vi "3_Case_loop.vi"() -> ()   [LabVIEW 2019]
uses:
  Instance           1 17Saved   Case_loop .vi
panel:
  in  "Enum":T1(ring) caption="Funkcja"
  out "?":bool
  out "?":bool
  out "?":bool=TRUE
  out "?":bool
  out "?":bool
  out "?":bool
  in  "Opóznienie [s]":dbl=0.009999999999999997 caption="Delay Time (s)" min=0.0 step=0.01 format="%#.2g"
  out "Waveform Chart":dynamicdata(graph)=[{"t0"=timestamp(3254228964.578125 s since 1904-01-01), "dt"=1.0, "Y"=[-0.9998476951563912]}, {"t0"=timestamp(3254228964.578125 s since 1904-01-01), "dt"=1.0, "Y"=[0.0]}]
  out "Numer iteracji":dbl=1709.0
  in  "?":bool
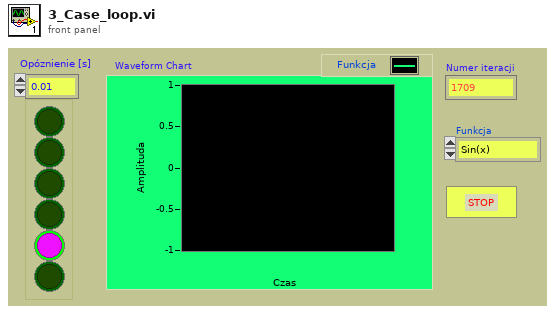
[diagram p1: front panel]
types:
  T1 = enum16{"Sin(x)", "Sin(x)+Cos(x)", "Sin(x)/x", "Sin(x)-Sin(2x)"}
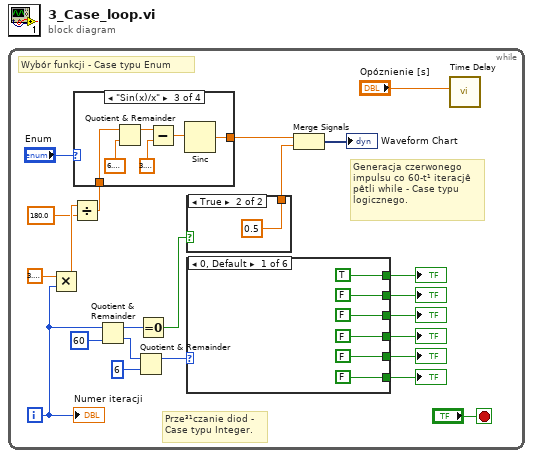
[diagram p0: block diagram]
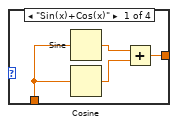
[diagram p2: hidden frame]
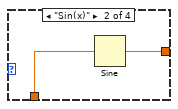
[diagram p3: hidden frame]
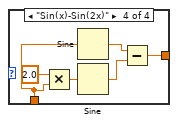
[diagram p4: hidden frame]
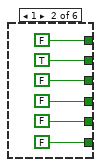
[diagram p5: hidden frame]
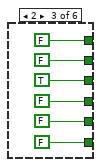
[diagram p6: hidden frame]
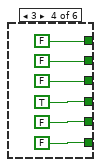
[diagram p7: hidden frame]
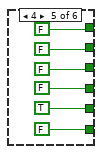
[diagram p8: hidden frame]
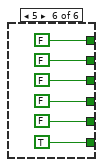
[diagram p9: hidden frame]
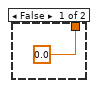
[diagram p10: hidden frame]
diagram:
  n1 = while {
    i -> [w11]
    stop <- "?" stop-if-true
    # "Wybór funkcji - Case typu Enum"
    # "Prze³¹czanie diod -\nCase typu Integer."
    # "Generacja czerwonego\nimpulsu co 60-t¹ iteracjê\npêtli while - Case typu \nlogicznego."
    n2 = Multiply(x=3.141592653589793, y=w11) -> (x*y=w13:dbl)
    n3 = Divide(x=w13, y=180.0) -> (x/y=w1:dbl)
    n4 = case shown="\"Sin(x)/x\"" "Enum" {
      tunnel: [w24 w29 w35 w41] -> w3
      tunnel: w1 -> [w27 w28 w30 w38]
      frame "Sin(x)+Cos(x)" {
        n5 = Sine(x=w27) -> (sin(x)=w25:dbl)
        n6 = Cosine(x=w27) -> (cos(x)=w26:dbl)
        n7 = Add(x=w25, y=w26) -> (x+y=w24:dbl)
      }
      frame "Sin(x)" {
        n8 = Sine(x=w28) -> (sin(x)=w29:dbl)
      }
      frame "Sin(x)/x" {
        n9 = Quotient & Remainder(x=w30, y=6.283185307179586) -> (x-y*floor(x/y)=w33:dbl)  [unwired: 1 out]
        n10 = Subtract(x=w33, y=3.141592653589793) -> (x-y=w31:dbl)
        n11 = Sinc(1:w31) -> (0:w35:dbl)
      }
      frame "Sin(x)-Sin(2x)" {
        n12 = Multiply(x=2.0, y=w38) -> (x*y=w37:dbl)
        n13 = Sine(x=w38) -> (sin(x)=w39:dbl)
        n14 = Sine(x=w37) -> (sin(x)=w40:dbl)
        n15 = Subtract(x=w39, y=w40) -> (x-y=w41:dbl)
      }
    }
    n16 = Quotient & Remainder(x=w11, y=60) -> (x-y*floor(x/y)=w9:i32, floor(x/y)=w8:i32)
    n17 = Quotient & Remainder(x=w8, y=6) -> (x-y*floor(x/y)=w6:i32)  [unwired: 1 out]
    n18 = Equal To 0?(x=w9) -> (x = 0?=w21:bool)
    n19 = case shown="True" w21 {
      tunnel: [0.0 ("x") 0.5 ("y")] -> w2
      frame False {
      }
      frame True {
      }
    }
    n20 = case shown="0, Default" w6 {
      tunnel: [FALSE ("Boolean") FALSE ("Boolean") FALSE ("Boolean") FALSE ("Boolean") FALSE ("Boolean") TRUE ("Boolean")] -> w20
      tunnel: [FALSE ("Boolean") FALSE ("Boolean") FALSE ("Boolean") FALSE ("Boolean") TRUE ("Boolean") FALSE ("Boolean")] -> w19
      tunnel: [FALSE ("Boolean") FALSE ("Boolean") FALSE ("Boolean") TRUE ("Boolean") FALSE ("Boolean") FALSE ("Boolean")] -> w18
      tunnel: [FALSE ("Boolean") FALSE ("Boolean") TRUE ("Boolean") FALSE ("Boolean") FALSE ("Boolean") FALSE ("Boolean")] -> w17
      tunnel: [FALSE ("Boolean") TRUE ("Boolean") FALSE ("Boolean") FALSE ("Boolean") FALSE ("Boolean") FALSE ("Boolean")] -> w16
      tunnel: [TRUE ("Boolean") FALSE ("Boolean") FALSE ("Boolean") FALSE ("Boolean") FALSE ("Boolean") FALSE ("Boolean")] -> w15
      frame 0, Default {
      }
      frame 1 {
      }
      frame 2 {
      }
      frame 3 {
      }
      frame 4 {
      }
      frame 5 {
      }
    }
    "?" <- w20
    "?" <- w19
    "?" <- w18
    "?" <- w17
    "?" <- w16
    "?" <- w15
    n21 = Merge Signals(w3, w2) -> (→"Waveform Chart":dynamicdata)
    n22 = call "Time Delay"("Delay Time (s)"="Opóznienie [s]") -> ()  [unwired: 10 in, 1 out]
    "Numer iteracji" <- w11
  }
